vi "MainVI.vi"() -> ()   [LabVIEW 2013]
panel:
  in  "Stop Button":bool
  out "Added?":string
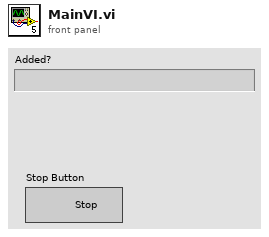
[diagram p1: front panel]
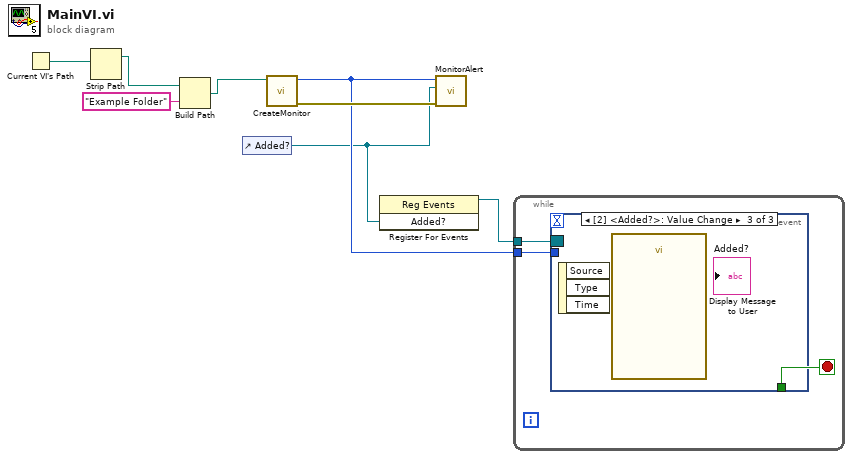
[diagram p0: block diagram]
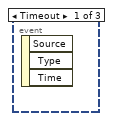
[diagram p2: hidden frame]
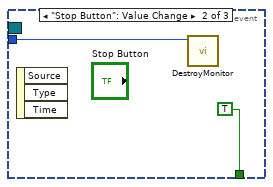
[diagram p3: hidden frame]
diagram:
  n1 = Current VI's Path() -> (path=w4:path)
  n2 = Strip Path(path=w4) -> (stripped path=w3:path)  [unwired: 1 out]
  n3 = Build Path(base path=w3, name or relative path="Example Folder") -> (appended path=w2:path)
  n4 = control-ref of="Added?"() -> (w6:refnum<vi>)
  n5 = call "CreateMonitor.vi"("File Path Control"=w2) -> ("error out"=w8:errorcluster, "Handle"=w7:i32)  [unwired: 9 in]
  n6 = register-events(w6) -> (reference out=w5:refnum<event-registration>)  [unwired: 2 in, 1 out]
  n7 = call "MonitorAlert.vi"("error in (no error)"=w8, "Str Refnum"=w6, "Handle"=w7) -> ()  [unwired: 8 in, 1 out]
  n8 = while {
    tunnel: w7 -> [w10]
    tunnel: w5 -> [w9]
    stop <- w11 stop-if-true
    n9 = event shown="[2] <Added?>: Value Change" {
      selector: w9 -> [_ _ _]
      dyn-events: _ -> [_ _ _]
      timeout: _ -> [_ _ _]
      tunnel: [_ TRUE _] -> w11
      tunnel: w10 -> [_ w12 _]
      event Timeout {
        n10 = event-data() -> ()  [unwired: 1 in, 3 out]
      }
      event "Stop Button": Value Change {
        n11 = event-data() -> ()  [unwired: 1 in, 3 out]
        n12 = call "DestroyMonitor.vi"("Handle in"=w12) -> ()  [unwired: 10 in, 1 out]
      }
      event Value Change {
        n13 = event-data() -> ()  [unwired: 1 in, 3 out]
        n14 = call "Display Message to User"() -> ()  [unwired: 10 in, 2 out]
      }
    }
  }
